vi "Controlword_ModeSpecific_Reference.vi"(10 "Operation Start":bool, 11 "ControlWord In":u16 format="%08b") -> (3 "ControlWord Out":u16 format="%08b")   [LabVIEW 2017, in "WordManipulationLibrary.lvlib"]
uses:
  WordManipulationLibrary.lvlib
  Bit Manipulation.lvlib
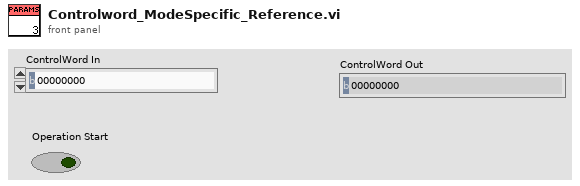
[diagram p1: front panel]
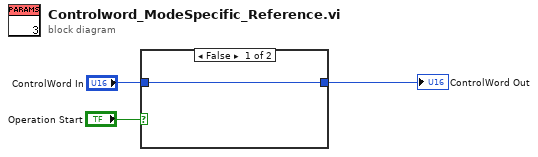
[diagram p0: block diagram]
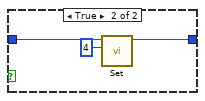
[diagram p2: hidden frame]
diagram:
  n1 = case shown="False" "Operation Start" {
    tunnel: "ControlWord In" -> [w4 w7]
    tunnel: [w4 w6] -> w2
    frame False {
    }
    frame True {
      n2 = call "Set.vi"("Bit to set"=u8 4, "Data_In"=w7) -> ("Data_Out"=w6:u16)  [unwired: 9 in]
    }
  }
  "ControlWord Out" <- w2
